vi "Add Actor.vi"(8 "error in":errorcluster, 11 "Target Item":T1) -> (0 "error out":errorcluster)   [LabVIEW 2023, in "Add Async Methods Actor.lvlib"]
uses:
  Add Async Methods Actor.lvlib
  <resource>/Framework/Providers/API/mxLvNIIM.ctl
  Classes/INI Store/INI Store.lvclass
  Classes/Target Store/Target Store.lvclass
  Localized Strings.vi
  AFPP Shared/AFPP Shared.lvlib
  C:/Users/AndreaVaccaro(LSInst/Downloads/Projects/Async Methods Actor/Providers/AddAsyncMethodsActor/Classes/Actor Store/Actor Store.lvclass
  C:/Users/AndreaVaccaro(LSInst/Downloads/Projects/Async Methods Actor/Providers/AddAsyncMethodsActor/Classes/INI Store/INI Store.lvclass
  C:/Users/AndreaVaccaro(LSInst/Downloads/Projects/Async Methods Actor/Providers/AddAsyncMethodsActor/Classes/Target Store/Target Store.lvclass
panel:
  out "Path Display":string
  in  "Path":path caption="Save files to..."
  in  "Remove Actor":bool
  in  "Inherit from:":string(combo)
  in  "Cancel Button":bool
  in  "OK Button":bool
  in  "Name of Actor":string
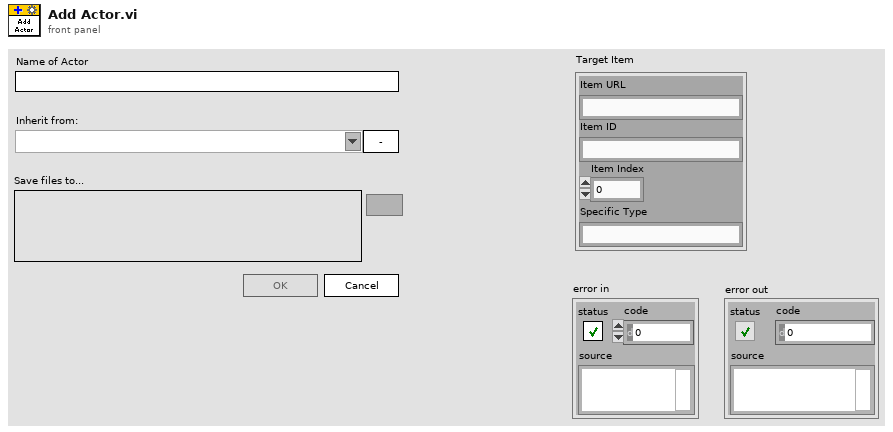
[diagram p1: front panel]
types:
  T1 = typedef "mxLvNIIM.ctl" = cluster{"Item URL":string, "Item ID":string, "Item Index":i32, "Specific Type":string}
  T2 = enum8{"Enabled", "Disabled", "Disabled and Grayed Out"}
  T3 = enum32{"Invalid", "Standard", "Closed", "Hidden", "Minimized", "Maximized"}
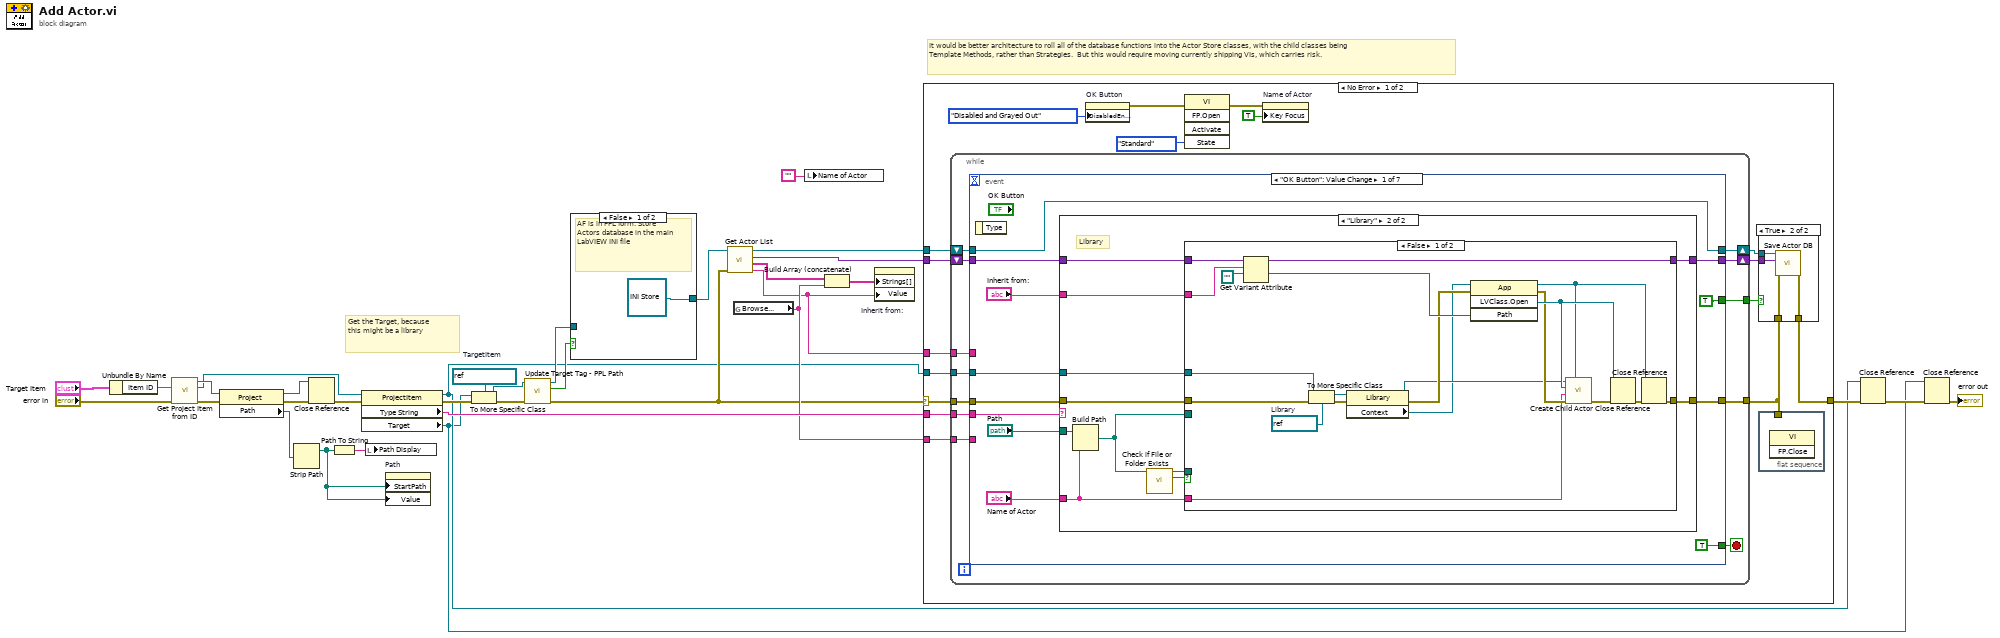
[diagram p0: block diagram]
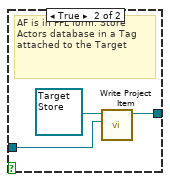
[diagram p2: hidden frame]
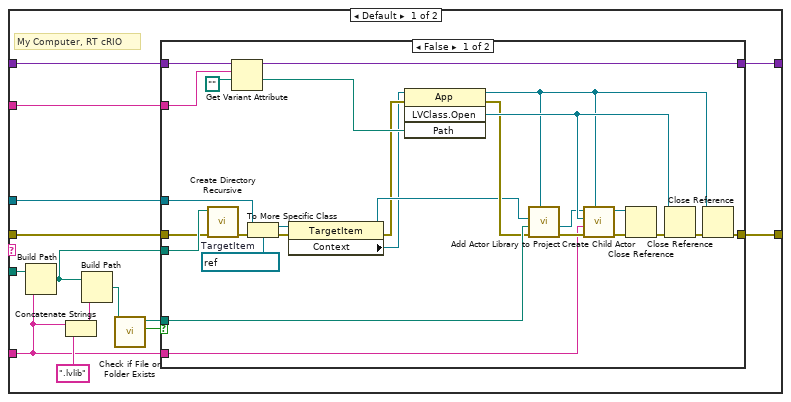
[diagram p3: hidden frame]
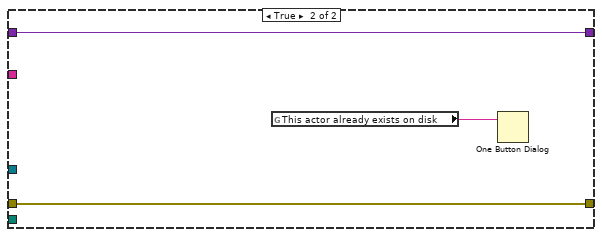
[diagram p4: hidden frame]
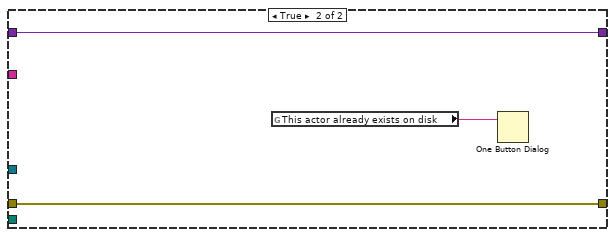
[diagram p5: hidden frame]
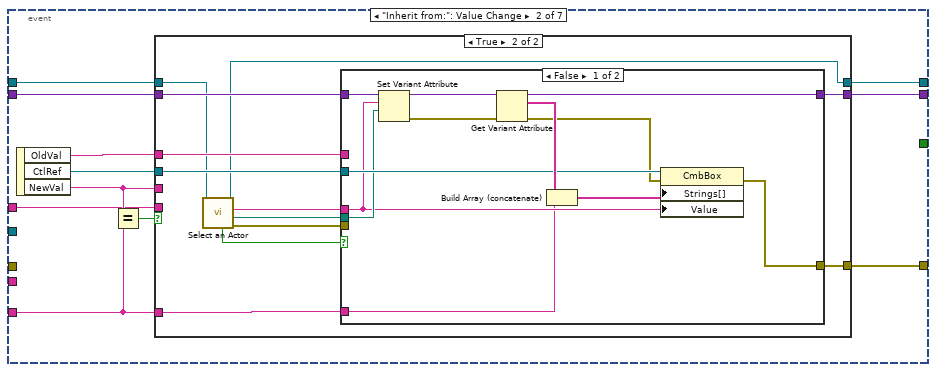
[diagram p6: hidden frame]
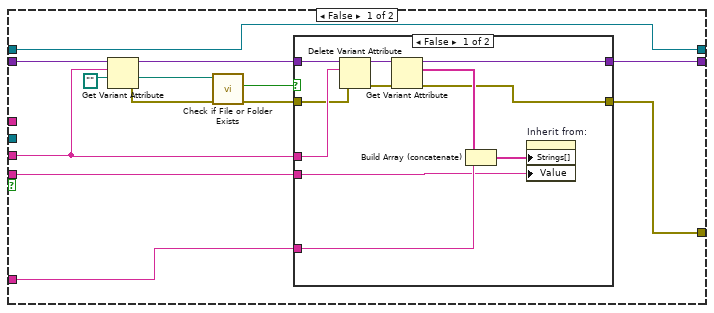
[diagram p7: hidden frame]
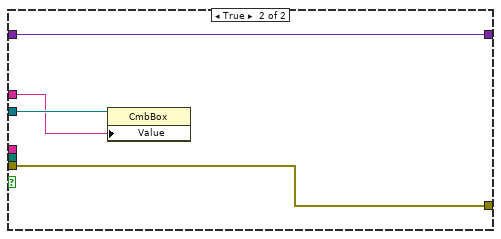
[diagram p9: hidden frame]
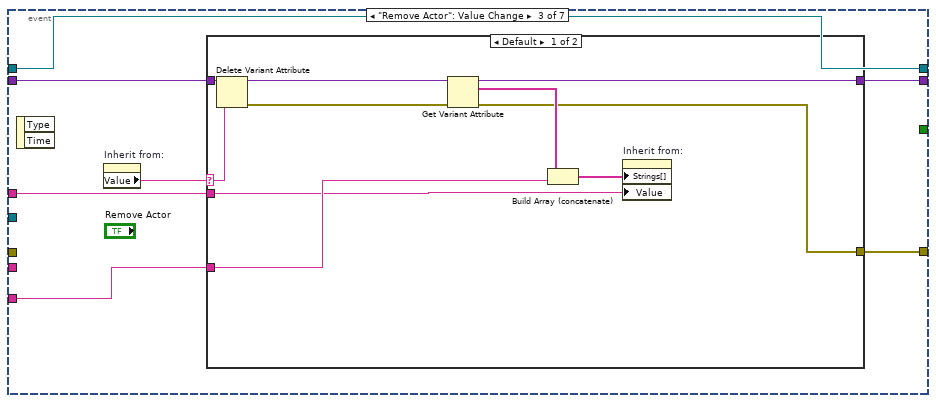
[diagram p10: hidden frame]
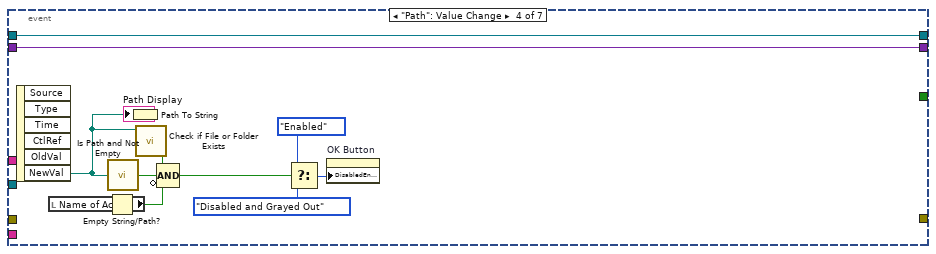
[diagram p12: hidden frame]
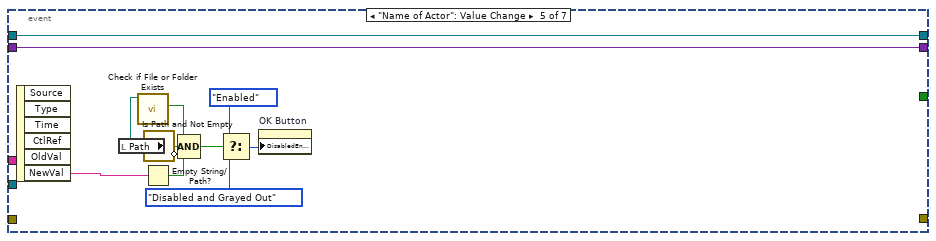
[diagram p13: hidden frame]
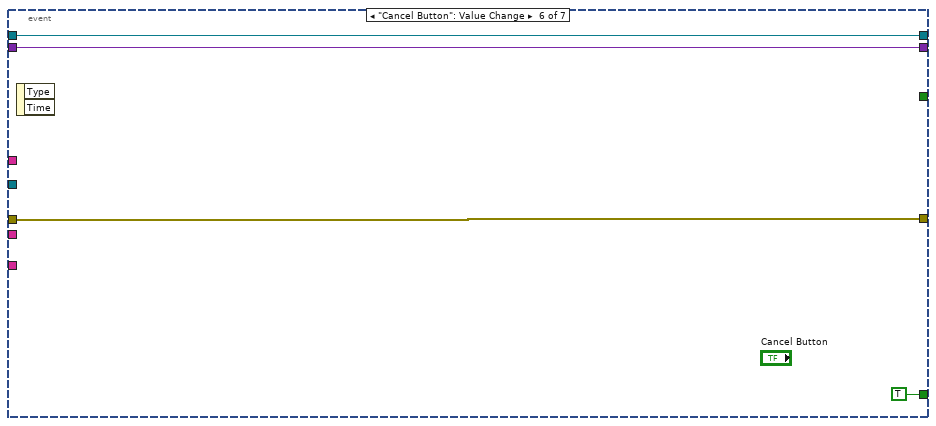
[diagram p14: hidden frame]
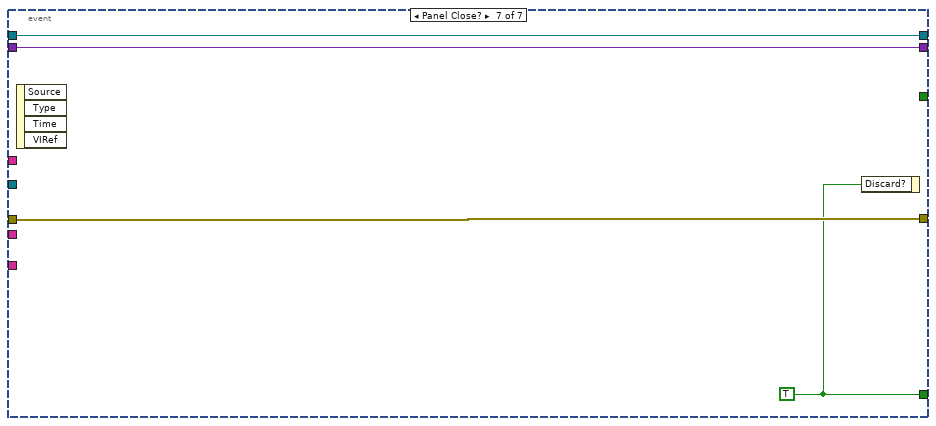
[diagram p15: hidden frame]
diagram:
  w8 = refnum<vi> refnum  # TargetItem
  # "Get the Target, because this might be a library"
  # "It would be better architecture to roll all of the database functions into the Actor Store classes, with the child classes being Template Methods, rather than Strategies.  But this would require moving currently shipping VIs, which carries risk."
  n1 = Unbundle By Name("Target Item") -> ("Item ID"=w1:string)
  n2 = call "Get Project Item from ID.vi"("error in (no error)"="error in", "Item ID"=w1) -> ("error out"=w27:errorcluster, "Project Item"=w23:refnum<vi>, "Project out"=w26:refnum<vi>)  [unwired: 7 in]
  n3 = property class="Project"(reference=w26, error in=w27) -> (reference out=w17:refnum<vi>, error out=w19:errorcluster, "Path"=w29:path)
  n4 = Strip Path(path=w29) -> (stripped path=w21:path)  [unwired: 1 out]
  n5 = Close Reference(reference=w17, error in (no error)=w19) -> (error out=w18:errorcluster)
  n6 = Path To String(path=w21) -> (string=w22:string)
  n7 = property class="ProjectItem"(reference=w23, error in=w18) -> (reference out=w3:refnum<vi>, error out=w5:errorcluster, "Type String"=w28:string, "Target"=w2:refnum<vi>)
  n8 = local write "Path Display"(w22) -> ()
  n9 = property on="Path" class="Path"("StartPath"=w21, "Value"=w21) -> ()  [unwired: 2 in, 2 out]
  n10 = To More Specific Class(target class=w8, reference=w2, error in=w5) -> (specific class reference=w7:refnum<vi>, error out=w6:errorcluster)
  n11 = call "Update Target Tag - PPL Path.vi"("error in (no error)"=w6, "Target"=w7) -> ("error out"=w9:errorcluster, "Found PPL?"=w16:bool, "dup Target"=w14:refnum<vi>)  [unwired: 7 in]
  n12 = case shown="False" w16 {
    tunnel: [refnum<class "INI Store.lvclass"> refnum ("Add Actor.lvlib:INI Store.lvclass") w37] -> w15
    tunnel: w14 -> [_ w35]
    frame False {
      # "AF is in PPL form. Store Actors database in the main LabVIEW INI file"
    }
    frame True {
      # "AF is in PPL form. Store Actors database in a Tag attached to the Target"
      n13 = call-dynamic "Write Project Item.vi"("Project Item"=w35, "Target Store in"=refnum<class "Target Store.lvclass"> refnum) -> ("Target Store out"=w37:refnum<class "Target Store.lvclass">)  [unwired: 9 in]
    }
  }
  n14 = call "Get Actor List.vi"("error in (no error)"=w9, "Actor Store"=w15) -> ("Actor Label"=w20:string, "Actors"=w12:string[], "Actor Paths"=w33:variant, "Actor Store"=w13:refnum<class "Actor Store.lvclass">)  [unwired: 6 in]
  n15 = global read "Localized Strings.vi" "Browse..."() -> (w24:string)
  n16 = local write "Name of Actor"("" ("Name of Actor")) -> ()
  n17 = Build Array (concatenate)(w12, w24) -> (w32:string[])
  n18 = property on="Inherit from:" class="CmbBox"("Strings[]"=w32, "Value"=w20) -> ()  [unwired: 2 in, 2 out]
  n19 = case shown="No Error" w9 {
    selector: w9 -> [w54 w276]
    tunnel: [w48 w276] -> w10
    tunnel: w33 -> [w53 _]
    tunnel: w28 -> [w52 _]
    tunnel: w3 -> [w51 _]
    tunnel: w24 -> [w50 _]
    tunnel: w20 -> [w46 _]
    tunnel: w13 -> [w45 _]
    frame No Error {
      n20 = while {
        tunnel: [w66] -> w42
        tunnel: w54 -> [w65]
        shift-right: [w62] -> w49
        shift-left: w53 -> [w63]
        tunnel: w52 -> [w61]
        tunnel: w51 -> [w60]
        tunnel: w50 -> [w59]
        tunnel: [w58] -> w47
        tunnel: w46 -> [w57]
        shift-right: [w55] -> w44
        shift-left: w45 -> [w56]
        stop <- w64 stop-if-true
        n21 = event shown="[0] \"OK Button\": Value Change" {
          selector: _ -> [_ _ _ _ _ _ _]
          dyn-events: _ -> [_ _ _ _ _ _ _]
          timeout: _ -> [_ _ _ _ _ _ _]
          tunnel: w65 -> [w72 _ _ _ _ w265 w270]
          tunnel: [w73 w167 w225 _ _ w265 w270] -> w66
          tunnel: [TRUE _ _ _ _ TRUE w268] -> w64
          tunnel: w63 -> [w76 w166 w227 w248 w255 w264 w269]
          tunnel: [w74 w165 w226 w248 w255 w264 w269] -> w62
          tunnel: w61 -> [w71 _ _ _ _ _ _]
          tunnel: w60 -> [w70 _ _ _ _ _ _]
          tunnel: w59 -> [_ w161 w224 _ _ _ _]
          tunnel: [TRUE _ _ _ _ _ _] -> w58
          tunnel: w57 -> [_ w160 w223 _ _ _ _]
          tunnel: w56 -> [w67 w158 w222 w240 w252 w263 w267]
          tunnel: [w67 w157 w222 w240 w252 w263 w267] -> w55
          event "OK Button": Value Change {
            n22 = event-data() -> ()  [unwired: 1 in, 1 out]
            n23 = case shown="\"Library\"" w71 {
              tunnel: "Path" -> [w92 w133]
              tunnel: "Name of Actor" -> [w80 w124]
              tunnel: w76 -> [w91 w132]
              tunnel: "Inherit from:" -> [w90 w131]
              tunnel: [w89 w130] -> w74
              tunnel: [w86 w128] -> w73
              tunnel: w72 -> [w85 w127]
              tunnel: w70 -> [w83 w125]
              frame Default {
                # "My Computer, RT cRIO"
                n24 = Build Path(base path=w92, name or relative path=w80) -> (appended path=w88:path)
                n25 = Concatenate Strings(w80, ".lvlib" ("string")) -> (w81:string)
                n26 = Build Path(base path=w88, name or relative path=w81) -> (appended path=w79:path)
                n27 = call <vilib>:"Check if File or Folder Exists.vi"("path"=w79) -> ("file or folder exists?"=w84:bool, "dup path"=w87:path)  [unwired: 8 in, 1 out]
                n28 = case shown="False" w84 {
                  tunnel: w80 -> [w103 _]
                  tunnel: w91 -> [w118 w122]
                  tunnel: w90 -> [w117 _]
                  tunnel: [w116 w122] -> w89
                  tunnel: w88 -> [w102 _]
                  tunnel: w87 -> [w113 _]
                  tunnel: [w104 w121] -> w86
                  tunnel: w85 -> [w101 w121]
                  tunnel: w83 -> [w107 _]
                  frame False {
                    w112 = refnum<vi> refnum  # TargetItem
                    n29 = call <vilib>:"Create Directory Recursive.vi"("error in (no error)"=w101, "directory"=w102) -> ("error out"=w100:errorcluster)  [unwired: 3 in, 2 out]
                    n30 = Get Variant Attribute(Variant=w118, name=w117, default value (empty Variant)=path "") -> (duplicate Variant=w116:variant, value=w115:path)  [unwired: 1 in, 2 out]
                    n31 = To More Specific Class(target class=w112, reference=w107, error in=w100) -> (specific class reference=w99:refnum<vi>, error out=w97:errorcluster)
                    n32 = property class="TargetItem"(reference=w99, error in=w97) -> (reference out=w98:refnum<vi>, error out=w96:errorcluster, "Context"=w95:refnum<vi>)
                    n33 = invoke class="App" method="LVClass.Open"(reference=w95, error in=w96, "Path"=w115) -> (reference out=w94:refnum<vi>, error out=w106:errorcluster, "LVClass.Open"=w119:refnum<vi>)  [unwired: 1 in, 1 out]
                    n34 = call "Add Actor Library to Project.vi"("Application"=w94, "error in (no error)"=w106, "Library Path"=w113, "Target Item"=w98) -> ("error out"=w111:errorcluster, "Library out"=w110:refnum<vi>)  [unwired: 6 in]
                    n35 = call "Create Child Actor.vi"("App Inst"=w94, "error in (no error)"=w111, "Actor Name"=w103, "Parent Class"=w119, "Library in"=w110) -> ("error out"=w109:errorcluster, "Library out"=w108:refnum<vi>)  [unwired: 5 in]
                    n36 = Close Reference(reference=w108, error in (no error)=w109) -> (error out=w93:errorcluster)
                    n37 = Close Reference(reference=w119, error in (no error)=w93) -> (error out=w105:errorcluster)
                    n38 = Close Reference(reference=w94, error in (no error)=w105) -> (error out=w104:errorcluster)
                  }
                  frame True {
                    n39 = global read "Localized Strings.vi" "This actor already exists on disk"() -> (w120:string)
                    n40 = One Button Dialog(message=w120) -> ()  [unwired: 1 in, 1 out]
                  }
                }
              }
              frame "Library" {
                # "Library"
                n41 = Build Path(base path=w133, name or relative path=w124) -> (appended path=w123:path)
                n42 = call <vilib>:"Check if File or Folder Exists.vi"("path"=w123) -> ("file or folder exists?"=w126:bool, "dup path"=w129:path)  [unwired: 8 in, 1 out]
                n43 = case shown="False" w126 {
                  tunnel: w124 -> [w142 _]
                  tunnel: w132 -> [w152 w156]
                  tunnel: w131 -> [w151 _]
                  tunnel: [w150 w156] -> w130
                  tunnel: w123 -> [_ _]
                  tunnel: w129 -> [_ _]
                  tunnel: [w143 w155] -> w128
                  tunnel: w127 -> [w141 w155]
                  tunnel: w125 -> [w146 _]
                  frame False {
                    w147 = refnum<vi> refnum  # Library
                    n44 = Get Variant Attribute(Variant=w152, name=w151, default value (empty Variant)=path "") -> (duplicate Variant=w150:variant, value=w149:path)  [unwired: 1 in, 2 out]
                    n45 = To More Specific Class(target class=w147, reference=w146, error in=w141) -> (specific class reference=w139:refnum<vi>, error out=w137:errorcluster)
                    n46 = property class="Library"(reference=w139, error in=w137) -> (reference out=w138:refnum<vi>, error out=w140:errorcluster, "Context"=w136:refnum<vi>)
                    n47 = invoke class="App" method="LVClass.Open"(reference=w136, error in=w140, "Path"=w149) -> (reference out=w135:refnum<vi>, error out=w145:errorcluster, "LVClass.Open"=w153:refnum<vi>)  [unwired: 1 in, 1 out]
                    n48 = call "Create Child Actor.vi"("App Inst"=w135, "error in (no error)"=w145, "Actor Name"=w142, "Parent Class"=w153, "Library in"=w138) -> ("error out"=w134:errorcluster)  [unwired: 5 in, 1 out]
                    n49 = Close Reference(reference=w153, error in (no error)=w134) -> (error out=w144:errorcluster)
                    n50 = Close Reference(reference=w135, error in (no error)=w144) -> (error out=w143:errorcluster)
                  }
                  frame True {
                    n51 = global read "Localized Strings.vi" "This actor already exists on disk"() -> (w154:string)
                    n52 = One Button Dialog(message=w154) -> ()  [unwired: 1 in, 1 out]
                  }
                }
              }
            }
          }
          event "Inherit from:": Value Change {
            n53 = event-data() -> ("OldVal"=w159:string, "CtlRef"=w164:refnum<vi>, "NewVal"=w162:string)  [unwired: 1 in]
            n54 = Equal?(x=w162, y=w161) -> (x = y?=w163:bool)
            n55 = case shown="True" w163 {
              tunnel: [w173 w199] -> w167
              tunnel: w166 -> [w180 w201]
              tunnel: [w174 w200] -> w165
              tunnel: w164 -> [_ w198]
              tunnel: w162 -> [w171 _]
              tunnel: w161 -> [w170 w197]
              tunnel: w160 -> [w169 _]
              tunnel: w159 -> [_ w196]
              tunnel: w158 -> [w168 w195]
              tunnel: [w168 w194] -> w157
              frame False {
                n56 = Get Variant Attribute(Variant=w180, name=w171, default value (empty Variant)=path "") -> (duplicate Variant=w177:variant, value=w179:path, error out=w176:errorcluster)  [unwired: 1 in, 1 out]
                n57 = call <vilib>:"Check if File or Folder Exists.vi"("error in (no error)"=w176, "path"=w179) -> ("error out"=w175:errorcluster, "file or folder exists?"=w172:bool)  [unwired: 7 in, 1 out]
                n58 = case shown="False" w172 {
                  tunnel: w177 -> [w191 w193]
                  tunnel: w171 -> [w190 _]
                  tunnel: w175 -> [w189 w192]
                  tunnel: [w184 w193] -> w174
                  tunnel: [w183 w192] -> w173
                  tunnel: w170 -> [w182 _]
                  tunnel: w169 -> [w181 _]
                  frame False {
                    n59 = Delete Variant Attribute(4:w189, 6:w190, 7:w191) -> (0:w185:errorcluster, 3:w188:variant)  [unwired: 1 out]
                    n60 = Get Variant Attribute(Variant=w188, error in=w185) -> (duplicate Variant=w184:variant, names=w186:string[], error out=w183:errorcluster)  [unwired: 2 in, 1 out]
                    n61 = Build Array (concatenate)(w186, w182) -> (w187:string[])
                    n62 = property on="Inherit from:" class="CmbBox"("Strings[]"=w187, "Value"=w181) -> ()  [unwired: 2 in, 2 out]
                  }
                  frame True {
                  }
                }
              }
              frame True {
                n63 = call "Select an Actor.vi"("Actor Store"=w195) -> ("error out"=w205:errorcluster, "Path to Actor"=w204:path, "Name of Actor"=w203:string, "Actor Store"=w194:refnum<class "Actor Store.lvclass">, "Cancelled"=w202:bool)  [unwired: 6 in]
                n64 = case shown="False" w202 {
                  tunnel: w203 -> [w207 _]
                  tunnel: w204 -> [w209 _]
                  tunnel: w205 -> [_ w220]
                  tunnel: w201 -> [w211 w221]
                  tunnel: [w214 w221] -> w200
                  tunnel: [w212 w220] -> w199
                  tunnel: w198 -> [w216 w219]
                  tunnel: w197 -> [w206 _]
                  tunnel: w196 -> [_ w218]
                  frame False {
                    n65 = Set Variant Attribute(Variant=w211, name=w207, value=w209) -> (Variant out=w210:variant, error out=w208:errorcluster)  [unwired: 1 in, 1 out]
                    n66 = Get Variant Attribute(Variant=w210, error in=w208) -> (duplicate Variant=w214:variant, names=w217:string[], error out=w213:errorcluster)  [unwired: 2 in, 1 out]
                    n67 = Build Array (concatenate)(w217, w206) -> (w215:string[])
                    n68 = property class="CmbBox"(reference=w216, error in=w213, "Strings[]"=w215, "Value"=w207) -> (error out=w212:errorcluster)  [unwired: 1 out]
                  }
                  frame True {
                    n69 = property class="CmbBox"(reference=w219, "Value"=w218) -> ()  [unwired: 1 in, 2 out]
                  }
                }
              }
            }
          }
          event "Remove Actor": Value Change {
            n70 = event-data() -> ()  [unwired: 1 in, 2 out]
            n71 = property on="Inherit from:" class="CmbBox"() -> ("Value"=w228:string)  [unwired: 2 in, 2 out]
            n72 = case shown="Default" w228 {
              selector: w228 -> [w234 _]
              tunnel: w227 -> [w237 w239]
              tunnel: [w236 w239] -> w226
              tunnel: [w235 _] -> w225
              tunnel: w224 -> [w230 _]
              tunnel: w223 -> [w229 _]
              frame Default {
                n73 = Delete Variant Attribute(6:w234, 7:w237) -> (0:w231:errorcluster, 3:w232:variant)  [unwired: 1 in, 1 out]
                n74 = Get Variant Attribute(Variant=w232, error in=w231) -> (duplicate Variant=w236:variant, names=w238:string[], error out=w235:errorcluster)  [unwired: 2 in, 1 out]
                n75 = Build Array (concatenate)(w238, w230) -> (w233:string[])
                n76 = property on="Inherit from:" class="CmbBox"("Strings[]"=w233, "Value"=w229) -> ()  [unwired: 2 in, 2 out]
              }
              frame "Actor", "Browse..." {
              }
            }
          }
          event "Path": Value Change {
            n77 = event-data() -> ("NewVal"=w241:path)  [unwired: 1 in, 5 out]
            n78 = local read "Name of Actor"() -> (w247:string)
            n79 = Empty String/Path?(string/path=w247) -> (empty?=w246:bool)
            n80 = call <vilib>:"Is Path and Not Empty.vi"("path"=w241) -> ("Is Path and Not Empty?"=w245:bool)  [unwired: 4 in]
            n81 = Path To String(path=w241) -> (string=→"Path Display":string)
            n82 = call <vilib>:"Check if File or Folder Exists.vi"("path"=w241) -> ("file or folder exists?"=w242:bool)  [unwired: 8 in, 2 out]
            n83 = Compound Arithmetic op=AND(w242, w245, invert w246) -> (w244:bool)
            n84 = Select(t=T2."Enabled" ("Disabled"), s=w244, f=T2."Disabled and Grayed Out" ("Disabled")) -> (s? t:f=w250:T2)
            n85 = property on="OK Button" class="Bool"("DisabledEnum"=w250) -> ()  [unwired: 2 in, 2 out]
          }
          event "Name of Actor": Value Change {
            n86 = event-data() -> ("NewVal"=w256:string)  [unwired: 1 in, 5 out]
            n87 = local read "Path"() -> (w253:path)
            n88 = call <vilib>:"Check if File or Folder Exists.vi"("path"=w253) -> ("file or folder exists?"=w254:bool)  [unwired: 8 in, 2 out]
            n89 = Empty String/Path?(string/path=w256) -> (empty?=w259:bool)
            n90 = call <vilib>:"Is Path and Not Empty.vi"("path"=w253) -> ("Is Path and Not Empty?"=w258:bool)  [unwired: 4 in]
            n91 = Compound Arithmetic op=AND(w254, w258, invert w259) -> (w257:bool)
            n92 = Select(t=T2."Enabled" ("Disabled"), s=w257, f=T2."Disabled and Grayed Out" ("Disabled")) -> (s? t:f=w261:T2)
            n93 = property on="OK Button" class="Bool"("DisabledEnum"=w261) -> ()  [unwired: 2 in, 2 out]
          }
          event "Cancel Button": Value Change {
            n94 = event-data() -> ()  [unwired: 1 in, 2 out]
          }
          event Panel Close? {
            w268 = TRUE
            n95 = event-data() -> ()  [unwired: 1 in, 4 out]
            n96 = event-data("Discard?"=w268) -> ()  [unwired: 1 in, 1 out]
          }
        }
      }
      n97 = property on="OK Button" class="Bool"("DisabledEnum"=T2."Disabled and Grayed Out" ("Disabled")) -> (error out=w38:errorcluster)  [unwired: 2 in, 1 out]
      n98 = invoke class="VI" method="FP.Open"(error in=w38, "State"=T3."Standard") -> (error out=w40:errorcluster)  [unwired: 3 in, 4 out]
      n99 = property on="Name of Actor" class="Str"(error in=w40, "Key Focus"=TRUE) -> ()  [unwired: 1 in, 2 out]
      n100 = case shown="True" w47 {
        tunnel: w49 -> [_ w273]
        tunnel: [w271 w275] -> w48
        tunnel: w42 -> [w271 w274]
        tunnel: w44 -> [_ w272]
        frame False {
        }
        frame True {
          n101 = call "Save Actor DB.vi"("error in (no error)"=w274, "Actor DB"=w273, "Actor Store"=w272) -> ("error out"=w275:errorcluster)  [unwired: 6 in, 2 out]
        }
      }
      n102 = flat-sequence {
        tunnel: w42 -> [_]
        frame #0 {
          n103 = invoke class="VI" method="FP.Close"() -> ()  [unwired: 3 in, 3 out]
        }
      }
    }
    frame Error {
    }
  }
  n104 = Close Reference(reference=w3, error in (no error)=w10) -> (error out=w11:errorcluster)
  n105 = Close Reference(reference=w2, error in (no error)=w11) -> (error out=→"error out":errorcluster)
